vi "Teardown.vi"(6 "Error":errorcluster, 7 "BaseActor":refnum<class "BaseActor.lvclass">, 10 "TeardownLocation":T1, 11 "UnheardMessages":refnum<class "Message.lvclass">[](array[class])) -> (5 "BaseActor":refnum<class "BaseActor.lvclass">)   [LabVIEW 2020, in "jettl.lvlib" / "BaseActor.lvlib" / "BaseActor.lvclass"]
uses:
  BaseActor.lvclass
  BaseActor.lvclass/BaseActor.ctl
  TeardownLocation.ctl
  jettl.lvlib
  Message/Message.lvclass
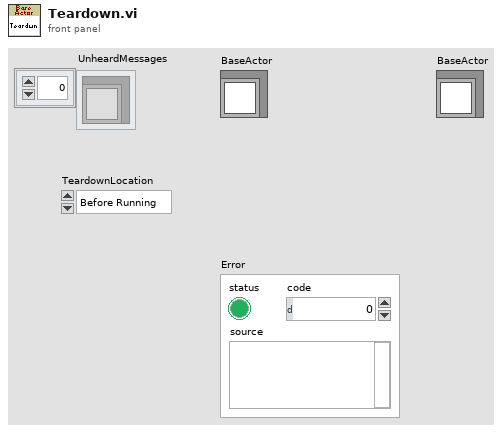
[diagram p1: front panel]
types:
  T1 = typedef "jettl.lvlib/TeardownLocation.ctl" = enum16{"Before Running", "After Running"}
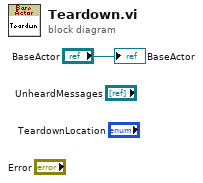
[diagram p0: block diagram]
diagram:
  "BaseActor" <- "BaseActor"
